vi "Close.vi"(8 "error in":errorcluster, 9 "timeout (-1)":i32=-1, 11 "Standard Engine Runtime in":refnum<class "Standard Engine Runtime.lvclass">) -> (0 "error out":errorcluster)   [LabVIEW 2013, in "Standard Engine Runtime.lvclass"]
doc: "This VI halts the execution of the engine background process and closes any references to it. The 'Stop' method should be called first so that the engine background process has a chance to properly uninitialize itself."
uses:
  Standard Engine Runtime.lvclass
  <vilib>/NI/Module Execution Interface/Engine Runtime/Execution States.ctl
  Standard Engine Runtime.lvclass/Standard Engine Runtime.ctl
  worker library/worker pool.lvlib
  <vilib>/NI/Module Execution Interface/Engine Runtime/Engine Runtime Interface.lvclass
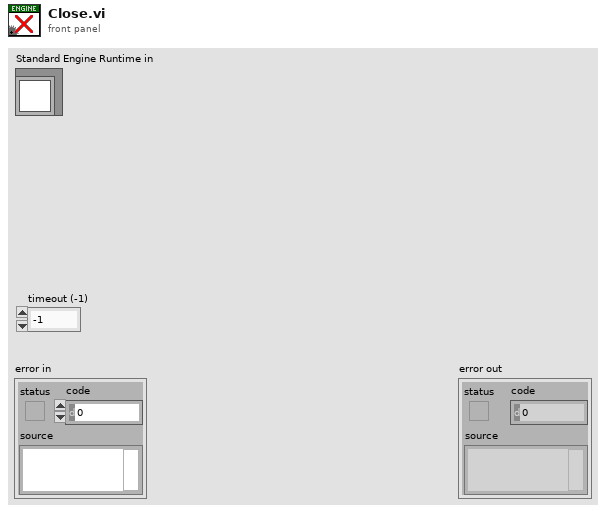
[diagram p1: front panel]
types:
  T1 = typedef "Engine Runtime Interface.lvclass/Execution States.ctl" = enum16{"Init", "Pre-Operational", "Safe-Operational", "Operational", "Stopped"}
  T2 = typedef "worker pool.lvlib/worker library reference.ctl" = cluster{"pool":refnum<vi>[], "worker comms":T3}
  T3 = typedef "worker pool.lvlib/worker comms.ctl" = cluster{"command fifo":refnum<k33>, "request fifos":T4, "response fifos":T5, "fault list":refnum<data-value>}
  T4 = typedef "worker pool.lvlib/request fifos.ctl" = cluster{"recovery":refnum<k33>, "fault fifo":refnum<k33>}
  T5 = typedef "worker pool.lvlib/response fifos.ctl" = cluster{"recovery":refnum<k33>}
  T6 = enum32{"Bad", "Idle", "Run top level", "Running"}
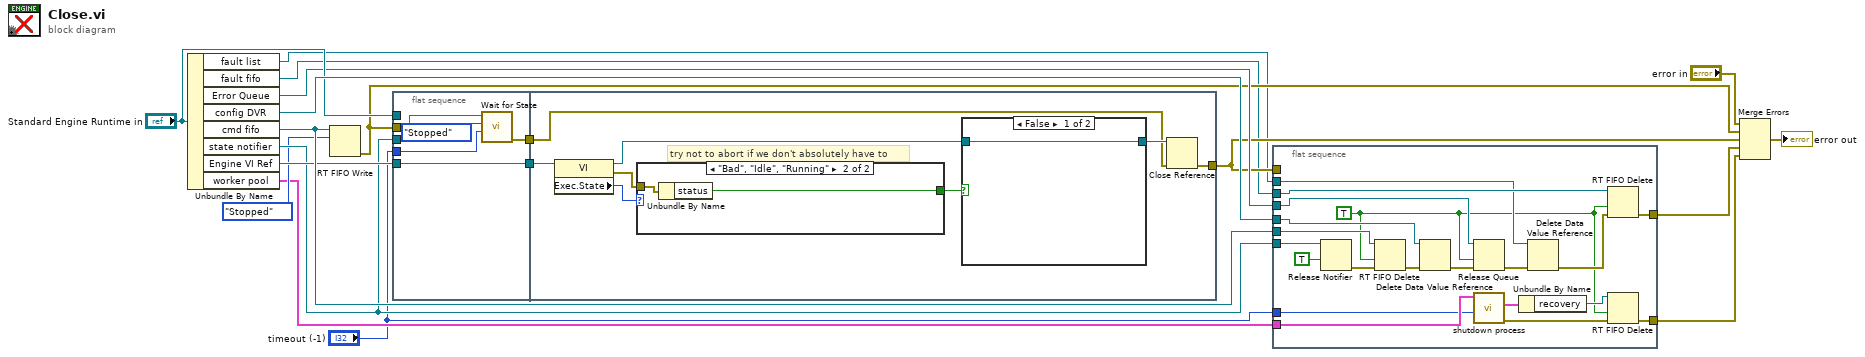
[diagram p0: block diagram]
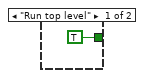
[diagram p2: hidden frame]
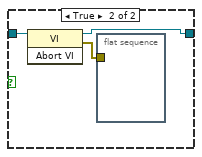
[diagram p3: hidden frame]
diagram:
  n1 = Unbundle By Name("Standard Engine Runtime in") -> ("fault list"=w1:refnum<data-value>, "fault fifo"=w2:refnum<k33>, "Error Queue"=w13:refnum<queue>, "config DVR"=w18:refnum<data-value>, "cmd fifo"=w19:refnum<k33>, "state notifier"=w7:refnum<notifier>, "Engine VI Ref"=w10:refnum<vi>, "worker pool"=w4:T2)
  n2 = RT FIFO Write(0:w19, 1:Execution_States."Stopped" ("element")) -> (11:w12:errorcluster)  [unwired: 3 in, 3 out]
  n3 = flat-sequence {
    tunnel: "Standard Engine Runtime in" -> [_]
    tunnel: w12 -> [_]
    tunnel: [w24] -> w11
    tunnel: w10 -> [w24]
    tunnel: [w23] -> w9
    tunnel: "timeout (-1)" -> [w22]
    tunnel: w7 -> [w21]
    tunnel: w11 -> [w32]
    tunnel: w9 -> [w26]
    tunnel: [w25] -> w8
    frame #0 {
      n4 = call "Wait for State.vi"("timeout in ms"=w22, "desired state"=Execution_States."Stopped", "state notifier"=w21) -> ("error out"=w23:errorcluster)  [unwired: 8 in]
    }
    frame #1 {
      # "try not to abort if we don't absolutely have to"
      n5 = property class="VI"(reference=w32) -> (reference out=w30:refnum<vi>, error out=w28:errorcluster, "Exec.State"=w29:T6)  [unwired: 1 in]
      n6 = case shown="\"Bad\", \"Idle\", \"Running\"" w29 {
        tunnel: w28 -> [_ w35]
        tunnel: [TRUE ("status") w34] -> w31
        frame "Run top level" {
        }
        frame "Bad", "Idle", "Running" {
          n7 = Unbundle By Name(w35) -> ("status"=w34:bool)
        }
      }
      n8 = case shown="False" w31 {
        tunnel: w30 -> [w36 w39]
        tunnel: [w36 w37] -> w27
        frame False {
        }
        frame True {
          n9 = invoke class="VI" method="Abort VI"(reference=w39) -> (reference out=w37:refnum<vi>, error out=w38:errorcluster)  [unwired: 2 in, 1 out]
          n10 = flat-sequence {
            tunnel: w38 -> [_]
            frame #0 {
            }
          }
        }
      }
      n11 = Close Reference(reference=w27, error in (no error)=w26) -> (error out=w25:errorcluster)
    }
  }
  n12 = flat-sequence {
    tunnel: w19 -> [w59]
    tunnel: w18 -> [w57]
    tunnel: w7 -> [w55]
    tunnel: [w43] -> w14
    tunnel: w13 -> [w51]
    tunnel: w8 -> [_]
    tunnel: [w46] -> w5
    tunnel: w4 -> [w49]
    tunnel: "timeout (-1)" -> [w48]
    tunnel: w2 -> [w42]
    tunnel: w1 -> [w41]
    frame #0 {
      w40 = TRUE ("force destroy? (F)")
      n13 = Release Notifier(notifier=w55, force destroy? (F)=TRUE) -> (error out=w54:errorcluster)  [unwired: 1 in, 2 out]
      n14 = RT FIFO Delete(0:w59, 2:w40, 3:w54) -> (11:w58:errorcluster)
      n15 = Delete Data Value Reference(data value reference=w57, error in=w58) -> (error out=w53:errorcluster)  [unwired: 1 out]
      n16 = Release Queue(queue=w51, force destroy? (F)=w40, error in (no error)=w53) -> (error out=w52:errorcluster)  [unwired: 2 out]
      n17 = call "shutdown process.vi"("timeout (500 ms)"=w48, "worker library"=w49) -> ("error out"=w50:errorcluster, "response fifos"=w47:T5)  [unwired: 8 in]
      n18 = Unbundle By Name(w47) -> ("recovery"=w45:refnum<k33>)
      n19 = Delete Data Value Reference(data value reference=w41, error in=w52) -> (error out=w44:errorcluster)  [unwired: 1 out]
      n20 = RT FIFO Delete(0:w42, 2:w40, 3:w44) -> (11:w43:errorcluster)
      n21 = RT FIFO Delete(0:w45, 2:w40, 3:w50) -> (11:w46:errorcluster)
    }
  }
  n22 = Merge Errors("error in", w12, w8, w14, w5) -> (→"error out":errorcluster)
